vi "laser_activation_logic.vi"(1 "Arm System":bool, 2 "Safety System":bool[](array[boolean])) -> (0 "Laser":bool)   [LabVIEW 2023]
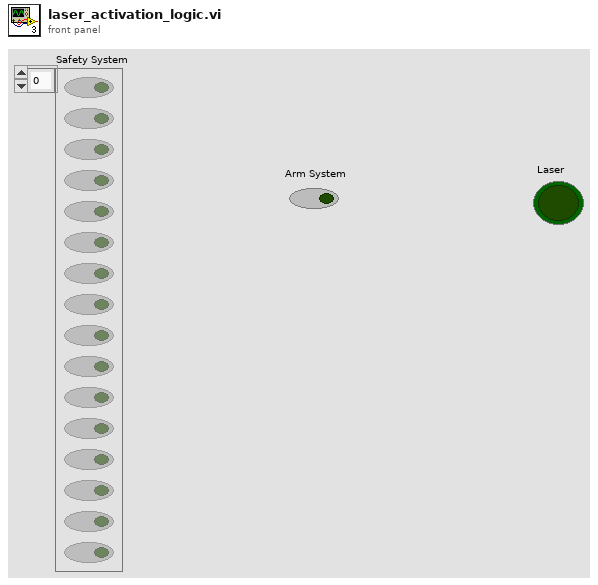
[diagram p1: front panel]
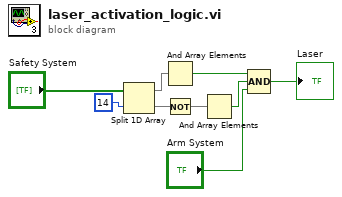
[diagram p0: block diagram]
diagram:
  n1 = Split 1D Array(array="Safety System", index=14) -> (first subarray=w5:bool[], second subarray=w8:bool[])
  n2 = And Array Elements(Boolean array=w5) -> (logical AND=w4:bool)
  n3 = Not(x=w8) -> (.not. x?=w3:bool[])
  n4 = And Array Elements(Boolean array=w3) -> (logical AND=w2:bool)
  n5 = Compound Arithmetic op=AND(w4, w2, "Arm System") -> (→"Laser":bool)
